vi "Log(by Ref).vi"(7 "Level":T1(ring), 8 "error in (no error)":errorcluster, 9 "error":errorcluster, 10 "Message":string, 11 "Logger Ref in":refnum<data-value>) -> (0 "error out":errorcluster, 3 "Logger Ref out":refnum<data-value>)   [LabVIEW 2017, in "Error Log.lvlib" / "Logger.lvclass"]
doc: "Creates a Record with the specified <b>Level</b>, <b>Message</b> and <b>error</b>, and passes it to the registered Handlers of the Logger pointed by the reference <b>Logger Ref in</B>."
uses:
  Logger.lvclass
  Logger.lvclass/Logger.ctl
  Get Handlers.vi
  Record.Error/Record.Error.lvclass
  \\192.168.1.40\Neosoft/Partage/Dossiers Personnels/BRO/DevTools_BR/wc/ErrorLog/src/Record/Record.lvclass
  Handler/Handler.lvclass
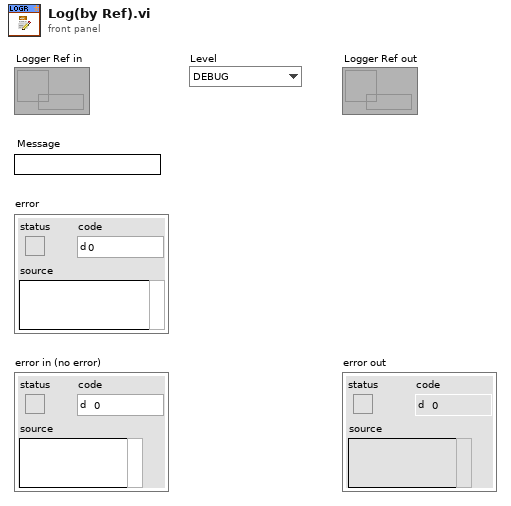
[diagram p1: front panel]
types:
  T1 = enum16{"DEBUG", "INFO", "WARNING", "ERROR", "CRITICAL"}
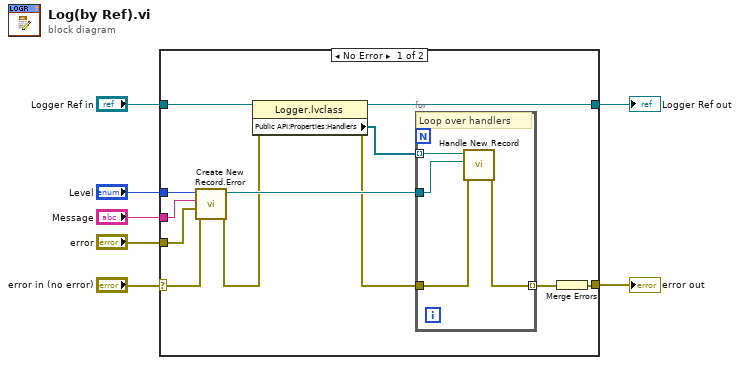
[diagram p0: block diagram]
diagram:
  n1 = case shown="No Error" "error in (no error)" {
    selector: "error in (no error)" -> [w15 w25]
    tunnel: [w13 w25] -> w6
    tunnel: [w11 w24] -> w1
    tunnel: "Logger Ref in" -> [w16 w24]
    tunnel: "Level" -> [w19 _]
    tunnel: "Message" -> [w18 _]
    tunnel: "error" -> [w17 _]
    frame No Error {
      n2 = call "Create New Record.Error.vi"("error in (no error)"=w15, "Error"=w17, "Message"=w18, "Level"=w19) -> ("error out"=w8:errorcluster, "Record.Error out"=w12:refnum<class "Record.Error.lvclass">)  [unwired: 6 in]
      n3 = property class="Logger.lvclass"(reference=w16, error in=w8) -> (reference out=w11:refnum<data-value>, error out=w9:errorcluster, "Public API:Properties:Handlers"=w10:refnum<class "Handler.lvclass">[])
      n4 = for {
        tunnel: w10 -> [w23] mode=indexing
        tunnel: w9 -> [w21]
        tunnel: [w20] -> w14 mode=indexing
        tunnel: w12 -> [w22]
        # "Loop over handlers"
        n5 = call "Handle New Record.vi"("error in (no error)"=w21, "New Record"=w22, "Handler in"=w23) -> ("error out"=w20:errorcluster)  [unwired: 7 in, 1 out]
      }
      n6 = Merge Errors(w14) -> (w13:errorcluster)
    }
    frame Error {
    }
  }
  "error out" <- w6
  "Logger Ref out" <- w1
